vi "AngleCorrection (2).vi"(8 "error in (no error)":errorcluster, 11 "Numeric in":dbl) -> (0 "error out":errorcluster, 3 "Numeric out":dbl)   [LabVIEW 2015]
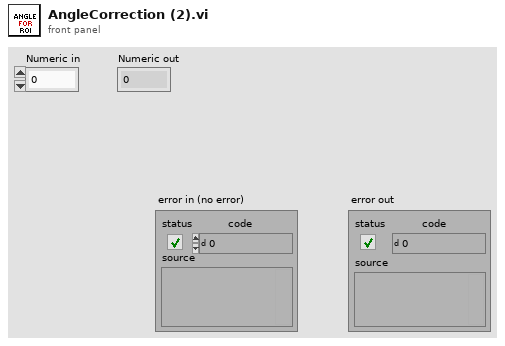
[diagram p1: front panel]
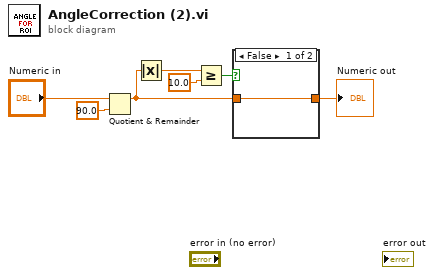
[diagram p0: block diagram]
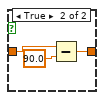
[diagram p2: hidden frame]
diagram:
  n1 = Quotient & Remainder(x="Numeric in", y=90.0) -> (x-y*floor(x/y)=w7:dbl)  [unwired: 1 out]
  n2 = Absolute Value(x=w7) -> (abs(x)=w5:dbl)
  n3 = Greater Or Equal?(x=w5, y=10.0) -> (x >= y?=w4:bool)
  n4 = case shown="False" w4 {
    tunnel: w7 -> [w8 w10]
    tunnel: [w8 w9] -> w3
    frame False {
    }
    frame True {
      n5 = Subtract(x=w10, y=90.0) -> (x-y=w9:dbl)
    }
  }
  "Numeric out" <- w3
